vi "Begin.vi"(8 "error in":errorcluster) -> (0 "error out":errorcluster)   [LabVIEW 2019]
doc: "Called before other user functions, this VI can be used to open I/O refnums, load in file data, and do general program initialization. Notice that the <B>error out</B> terminal is simply used for data flow. Wiring it to other structures or subVIs ensures that this VI runs first."
uses:
  <vilib>/Rock Robotics/WPI/DriverStation/WPI_DriverStationRobotMode2.ctl
  <vilib>/Rock Robotics/WPI/Joystick/WPI_JoystickDeviceEnum.ctl
  <vilib>/Rock Robotics/SystemInterfaces/DIO/FPGA_DIOPWMChannel.ctl
  <vilib>/Rock Robotics/WPI/SafetyOutput/WPI_SafetyOutputConfigMenu.ctl
  <vilib>/Rock Robotics/WPI/Solenoid/WPI_SolenoidChannel.ctl
  <vilib>/Rock Robotics/SystemInterfaces/i2clib/i2c_bus.ctl
  <vilib>/Rock Robotics/WPI/Solenoid/WPI_SolenoidValue.ctl
  Robot Global Data.vi
  <vilib>/Rock Robotics/WPI/RobotDrive/WPI_RobotDriveOpen2MotorWithExistingMotors.vi
  <vilib>/Rock Robotics/WPI/MotorControl/WPI_MotorControlOpen SPARK.vi
  <vilib>/Rock Robotics/WPI/Solenoid/WPI_SolenoidOpenDouble.vi
  <vilib>/Rock Robotics/WPI/Solenoid/WPI_SolenoidSetEnum.vi
  <vilib>/Rock Robotics/Network Tables/NT Write Number.vi
  <vilib>/Rock Robotics/Network Tables/NT Write Boolean Array.vi
  <vilib>/Rock Robotics/Network Tables/NT Write Numeric Array.vi
panel:
  in  "Blue Calibration":cluster{"R":dbl, "G":dbl, "B":dbl}={"R"=0.143, "G"=0.427, "B"=0.429}
  in  "Green Calibration":cluster{"R":dbl, "G":dbl, "B":dbl}={"R"=0.197, "G"=0.561, "B"=0.24}
  in  "Red Calibration":cluster{"R":dbl, "G":dbl, "B":dbl}={"R"=0.561, "G"=0.323, "B"=0.114}
  in  "Yellow Calibration":cluster{"R":dbl, "G":dbl, "B":dbl}={"R"=0.361, "G"=0.524, "B"=0.113}
  in  "Calibration Time (sec)":u32=4
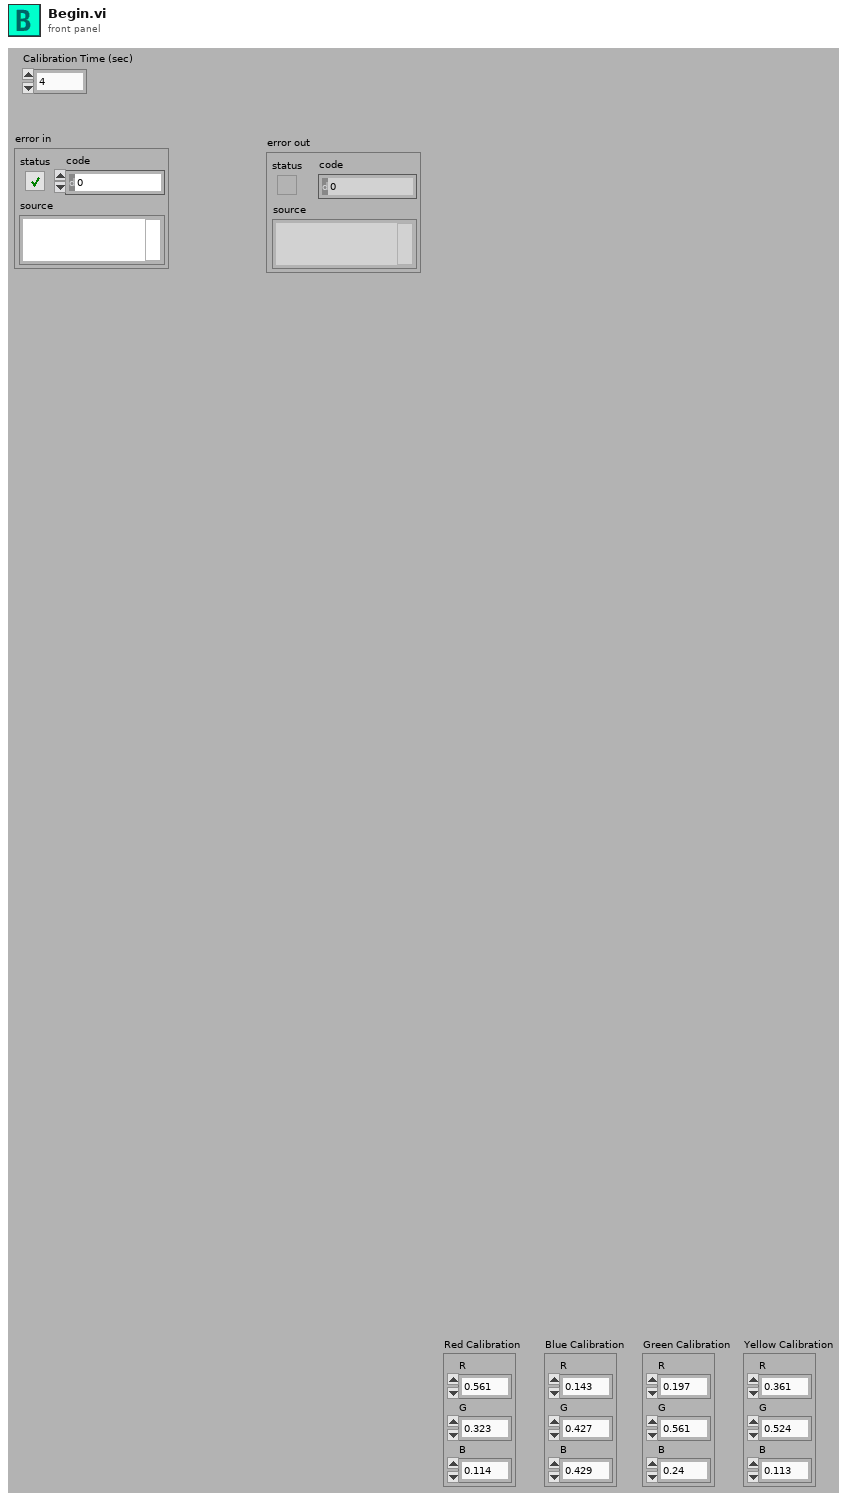
[diagram p1: front panel]
types:
  T1 = typedef "WPI_SolenoidChannel.ctl" = enum8{"Solenoid 0", "Solenoid 1", "Solenoid 2", "Solenoid 3", "Solenoid 4", "Solenoid 5", "Solenoid 6", "Solenoid 7", "Invalid"}
  T2 = typedef "WPI_SolenoidValue.ctl" = enum16{"Off", "On", "Forward", "Reverse"}
  T3 = typedef "WPI_SafetyOutputConfigMenu.ctl" = enum16{"Enable", "Disable"}
  T4 = typedef "i2c_bus.ctl" = enum16{"I2C On-Board", "I2C MXP", "Invalid"}
  T5 = typedef "FPGA_DIOPWMChannel.ctl" = enum8{"PWM 0", "PWM 1", "PWM 2", "PWM 3", "PWM 4", "PWM 5", "PWM 6", "PWM 7", "PWM 8", "PWM 9", "PWM MXP 0", "PWM MXP 1", "PWM MXP 2", "PWM MXP 3", "PWM MXP 4", "PWM MXP 5", "PWM MXP 6", "PWM MXP 7", "PWM MXP 8", "PWM MXP 9", "Invalid"}
  T6 = typedef "WPI_JoystickDeviceEnum.ctl" = enum16{"USB 0", "USB 1", "USB 2", "USB 3", "USB 4", "USB 5"}
  T7 = typedef "WPI_DriverStationRobotMode2.ctl" = enum16{"Autonomous Disabled", "Autonomous Enabled", "Teleop Disabled", "Teleop Enabled", "Disconnected", "Finish", "Test Disabled", "Test Enabled", "Emergency Stopped"}
  T8 = typedef "WPI_JoystickDevRef.ctl" = cluster{"Device":T6}
  T9 = typedef "WPI_MotorControlDeviceRef.ctl" = cluster{"DeviceStatus":errorcluster, "Type":T10, "PWM":cluster{"PWM Channel":T5, "DeadBand":T11}, "CAN":cluster{"Device Number":u8, "SetOutput VI Ref":variant, "GetOutput VI Ref":variant, "Enable VI Ref":variant, "Disable VI Ref":variant, "Data":variant}, "Invert":bool, "DIO PWM":cluster{"PWM \"Enable\" Channel":T5, "DIOChannel":T12, "PWM Rate":dbl}}
  T10 = typedef "WPI_MotorControlType.ctl" = enum16{"PWM", "CAN", "DIO PWM"}
  T11 = typedef "WPI_PWMDeadband.ctl" = cluster{"Name":string, "maxPositivePwm":i32, "minPositivePwm":i32, "centerPwm":i32, "maxNegativePwm":i32, "minNegativePwm":i32, "angularRange":u16}
  T12 = typedef "FPGA_DIOChannel.ctl" = enum8{"DIO 0", "DIO 1", "DIO 2", "DIO 3", "DIO 4", "DIO 5", "DIO 6", "DIO 7", "DIO 8", "DIO 9", "DIO MXP 0", "DIO MXP 1", "DIO MXP 2", "DIO MXP 3", "DIO MXP 4", "DIO MXP 5", "DIO MXP 6", "DIO MXP 7", "DIO MXP 8", "DIO MXP 9", "DIO MXP 10", "DIO MXP 11", "DIO MXP 12", "DIO MXP 13", "DIO MXP 14", "DIO MXP 15", "SPI Port CS1", "SPI Port CS2", "SPI Port CS3", "SPI Port MISO", "SPI Port MOSI", "Invalid"}
  T13 = typedef "WPI_RobotDriveDevRef.ctl" = cluster{"DevStatus":errorcluster, "Motors[]":T9[], "Square Inputs":bool, "Max Output":dbl}
  T14 = typedef "ADIS 16448 HW Configuration.ctl" = cluster{"SPI Clock Rate (Hz)":dbl, "IMU SPI Mode (3)":T15, "IMU Reset Pin":T12, "IMU SPI Bus":T16, "IMU Data Ready Pin":T12, "Stall Config":cluster{"Pow2BytesPerRead":u8, "StallTicks":u16, "CsToSclkTicks":u8}, "IMU Status LED Pin":T12}
  T15 = typedef "WPI_SPIMode.ctl" = enum16{"Mode 0 (Clk Idle Low,Sample on Leading)", "Mode 1 (Clk Idle Low,Sample on Trailing)", "Mode 2 (Clk Idle High,Sample on Leading)", "Mode 3 (Clk Idle High,Sample on Trailing)"}
  T16 = typedef "spi_bus.ctl" = enum16{"SPI On-Board, CS0", "SPI On-Board, CS1", "SPI On-Board, CS2", "SPI On-Board, CS3", "SPI MXP", "Invalid"}
  T17 = typedef "Color Sensor V3 DevRef.ctl" = cluster{"I2CDevRef":T18}
  T18 = typedef "WPI_I2CDevRef.ctl" = cluster{"DevStatus":errorcluster, "Device Address":u8, "Handle":i32, "I2C Bus":T4}
  T19 = typedef "WPI_SolenoidDevRef.ctl" = cluster{"DevStatus":errorcluster, "Pneumatics Control Module":u8, "Forward Solenoid Channel":T1, "Reverse Solenoid Channel":T1}
  T20 = typedef "ADIS16448 Device Reference.ctl" = cluster{"DevStatus":errorcluster, "Hardware Config":T21, "Calibration Complete":refnum<notifier>, "Status FIFO":refnum<k33>, "Last Value Reference":refnum<data-value>, "Sychronous Process VI":T22, "Cmd FIFO":refnum<k33>, "Source":T23, "Data FIFO":refnum<k33>, "IMU Status LED Pin":T12, "Calibration Time":u32}
  T21 = typedef "ADIS16448 Hardware Configuration.ctl" = cluster{"SPI Clock Rate (Hz)":dbl, "IMU SPI Mode (3)":T15, "IMU Reset Pin":T12, "IMU SPI Bus":T16, "IMU Data Ready Pin":T12, "Stall Config":cluster{"Pow2BytesPerRead":u8, "StallTicks":u16, "CsToSclkTicks":u8}, "IMU Status LED Pin":T12}
  T22 = typedef "ADIS16448 Process.ctl" = refnum<vi>
  T23 = typedef "FPGA_CounterEncoderSourceConvertionLVSourceType.ctl" = cluster{"DevStatus":errorcluster, "AnalogTriggerMode?":bool, "DigitalMode":cluster{"DIO Channel":T24}, "AnalogTriggerMode":cluster{"AnalogTriggerIndex":T25, "OutputType":T26}}
  T24 = typedef "FPGA_DIODigitalSourceChannel.ctl" = enum8{"DIO 0", "DIO 1", "DIO 2", "DIO 3", "DIO 4", "DIO 5", "DIO 6", "DIO 7", "DIO 8", "DIO 9", "DIO MXP 0", "DIO MXP 1", "DIO MXP 2", "DIO MXP 3", "DIO MXP 4", "DIO MXP 5", "DIO MXP 6", "DIO MXP 7", "DIO MXP 8", "DIO MXP 9", "DIO MXP 10", "DIO MXP 11", "DIO MXP 12", "DIO MXP 13", "DIO MXP 14", "DIO MXP 15", "SPI Port CS1", "SPI Port CS2", "SPI Port CS3", "SPI Port MISO", "SPI Port MOSI", "Disabled"}
  T25 = typedef "FPGA_AnalogTriggerIndex.ctl" = enum8{"Trig 0", "Trig 1", "Trig 2", "Trig 3", "Trig 4", "Trig 5", "Trig 6", "Trig 7", "Invalid"}
  T26 = typedef "FPGA_AnalogTriggerOutType.ctl" = enum16{"InWindow", "TriggerState", "Rising", "Falling"}
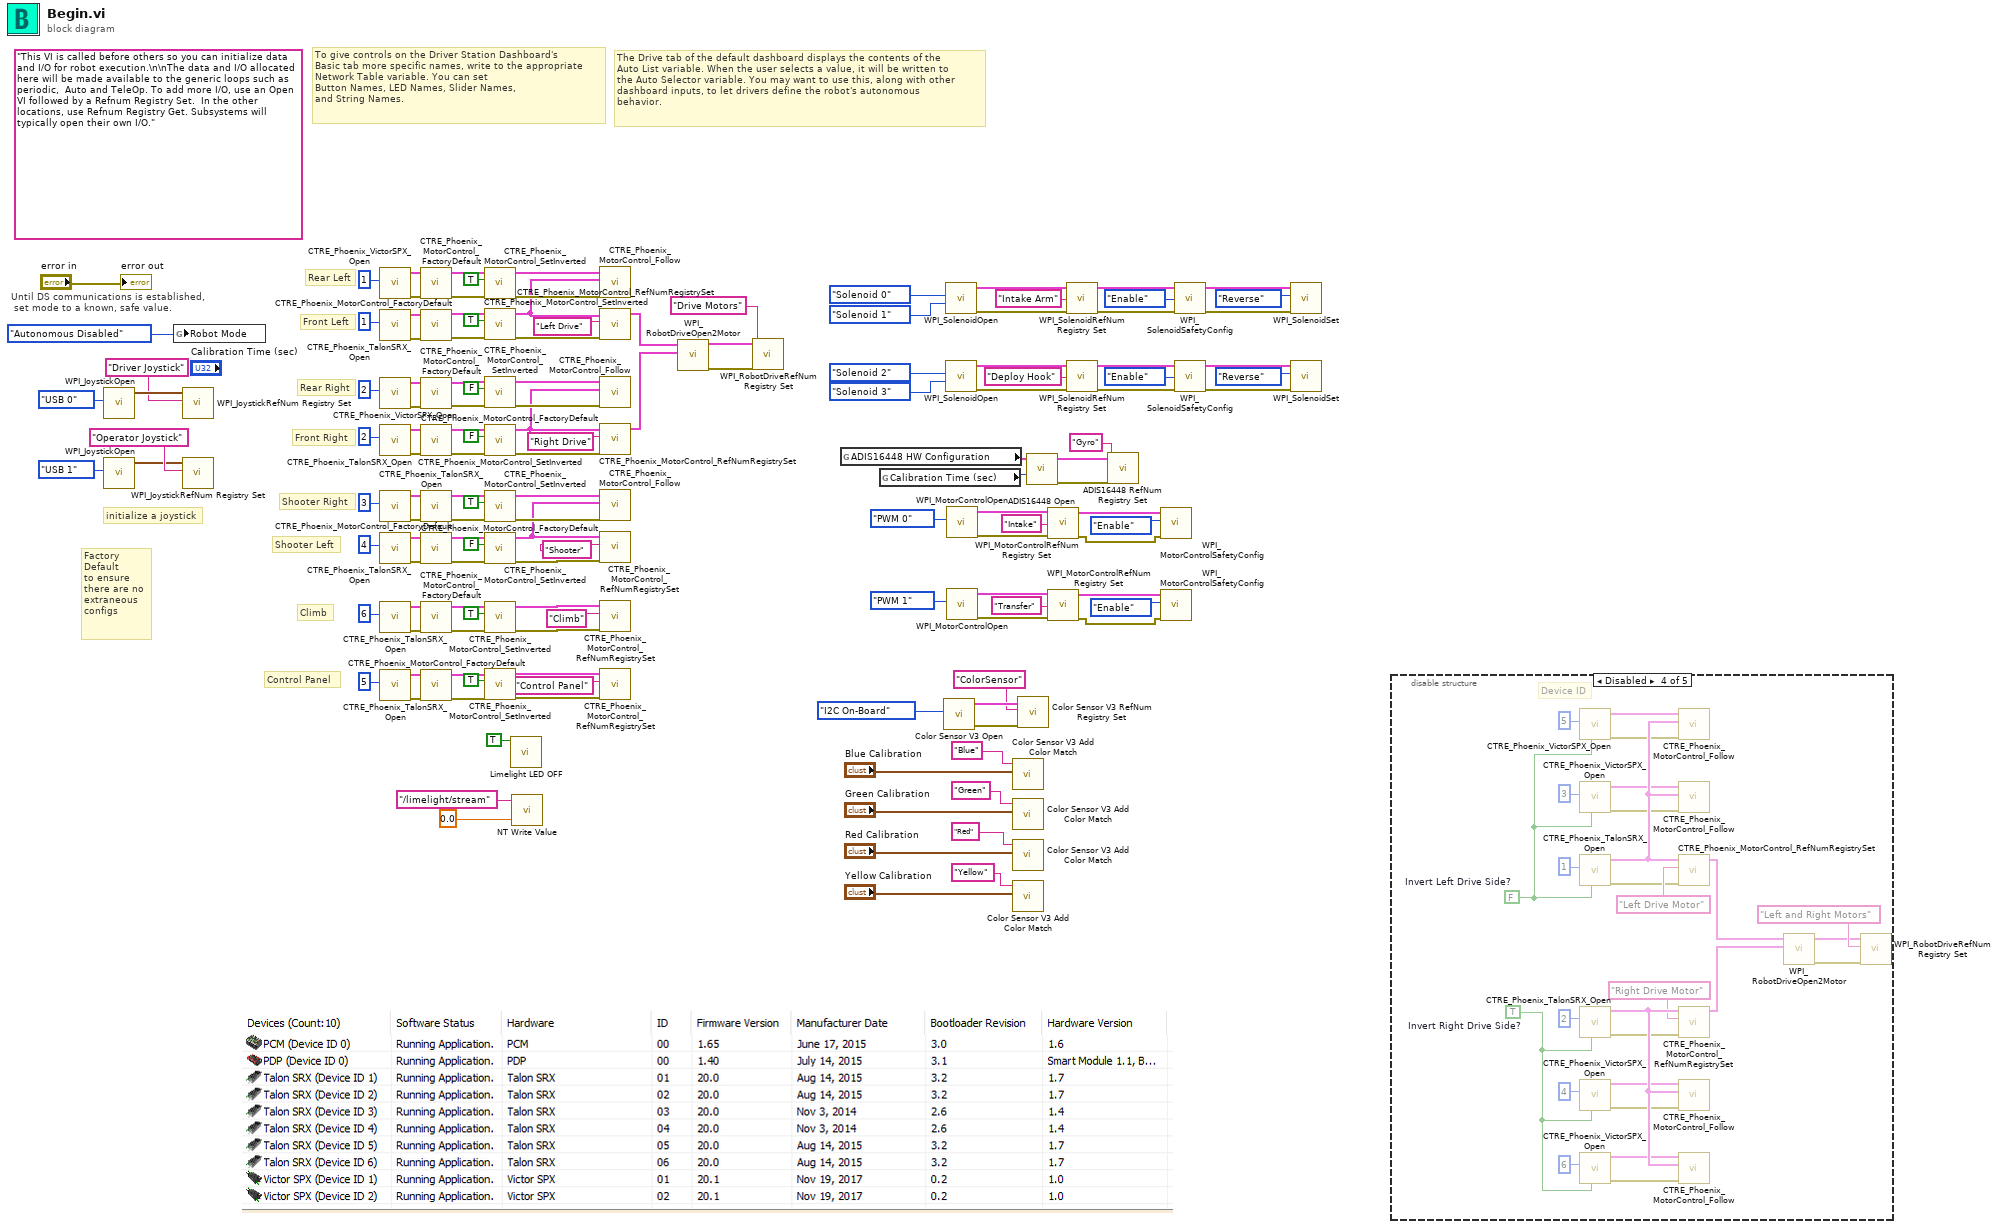
[diagram p0: block diagram]
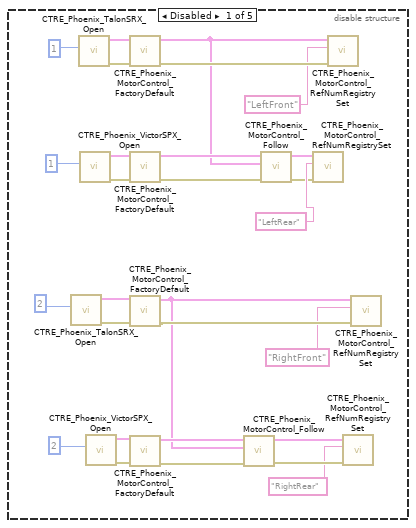
[diagram p2: hidden frame]
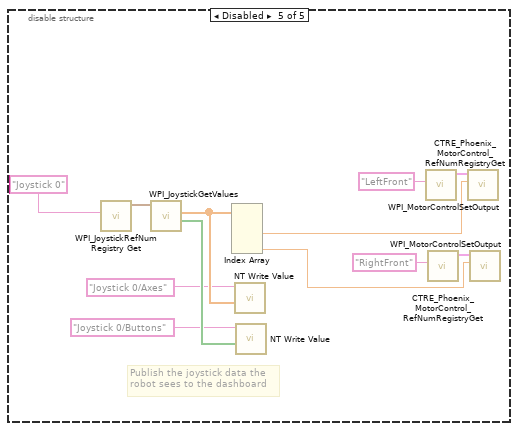
[diagram p5: hidden frame]
diagram:
  (unwired) "This VI is called before others so you can initialize data and I/O for robot execution.\n\nThe data and I/O allocated here will be made available to the generic loops such as periodic,  Auto and TeleOp. To add more I/O, use an Open VI followed by a Refnum Registry Set.  In the other locations, use Refnum Registry Get. Subsystems will typically open their own I/O."
  # "Climb"
  # "Control Panel"
  # "The Drive tab of the default dashboard displays the contents of the\nAuto List variable. When the user selects a value, it will be written to\nthe Auto Selector variable. You may want to use this, along with other\ndashboard inputs, to let drivers define the robot's autonomous\nbehavior."
  # "To give controls on the Driver Station Dashboard's\nBasic tab more specific names, write to the appropriate\nNetwork Table variable. You can set\nButton Names, LED Names, Slider Names,\nand String Names."
  # "Shooter Left"
  # "Shooter Right"
  # "Factory \nDefault \nto ensure \nthere are no \nextraneous \nconfigs"
  # "Front Right"
  # "Front Left"
  # "Rear Right"
  # "Rear Left"
  # "initialize a joystick"
  # "Until DS communications is established,\n set mode to a known, safe value."
  n1 = call <vilib>:"WPI_JoystickOpen.vi"("JoystickDevice"=WPI_JoystickDeviceEnum."USB 0") -> ("JoystickDevRef"=w121:T8)  [unwired: 10 in]
  n2 = call <vilib>:"WPI_JoystickOpen.vi"("JoystickDevice"=WPI_JoystickDeviceEnum."USB 1") -> ("JoystickDevRef"=w136:T8)  [unwired: 10 in]
  n3 = global write "Robot Global Data.vi" "Robot Mode"(WPI_DriverStationRobotMode2."Autonomous Disabled" ("Robot Mode")) -> ()
  n4 = call <vilib>:"WPI_JoystickRefNum Registry Set.vi"("refnum name"="Driver Joystick", "JoystickDevRef"=w121) -> ()  [unwired: 8 in, 2 out]
  n5 = call <vilib>:"WPI_JoystickRefNum Registry Set.vi"("refnum name"="Operator Joystick", "JoystickDevRef"=w136) -> ()  [unwired: 8 in, 2 out]
  n6 = call <vilib>:"CTRE_Phoenix_VictorSPX_Open.vi"("Device Number"=u8 1) -> ("error out"=w119:errorcluster, "CAN Talon SRX Ref"=w118:T9)  [unwired: 9 in]
  n7 = call <vilib>:"CTRE_Phoenix_TalonSRX_Open.vi"("Device Number"=u8 1) -> ("error out"=w116:errorcluster, "CAN Talon SRX Ref"=w117:T9)  [unwired: 9 in]
  n8 = call <vilib>:"CTRE_Phoenix_VictorSPX_Open.vi"("Device Number"=u8 2) -> ("error out"=w115:errorcluster, "CAN Talon SRX Ref"=w114:T9)  [unwired: 9 in]
  n9 = call <vilib>:"CTRE_Phoenix_TalonSRX_Open.vi"("Device Number"=u8 2) -> ("error out"=w113:errorcluster, "CAN Talon SRX Ref"=w112:T9)  [unwired: 9 in]
  n10 = call <vilib>:"CTRE_Phoenix_TalonSRX_Open.vi"("Device Number"=u8 3) -> ("error out"=w74:errorcluster, "CAN Talon SRX Ref"=w73:T9)  [unwired: 9 in]
  n11 = call <vilib>:"CTRE_Phoenix_TalonSRX_Open.vi"("Device Number"=u8 4) -> ("error out"=w72:errorcluster, "CAN Talon SRX Ref"=w71:T9)  [unwired: 9 in]
  n12 = call <vilib>:"CTRE_Phoenix_TalonSRX_Open.vi"("Device Number"=u8 6) -> ("error out"=w13:errorcluster, "CAN Talon SRX Ref"=w12:T9)  [unwired: 9 in]
  n13 = call <vilib>:"CTRE_Phoenix_TalonSRX_Open.vi"("Device Number"=u8 5) -> ("error out"=w47:errorcluster, "CAN Talon SRX Ref"=w46:T9)  [unwired: 9 in]
  n14 = call <vilib>:"CTRE_Phoenix_MotorControl_FactoryDefault.vi"("error in"=w119, "PhoenixMotorControlDevRef"=w118) -> ("error out"=w110:errorcluster, "PhoenixMotorControlDevRef"=w109:T9)  [unwired: 8 in]
  n15 = call <vilib>:"CTRE_Phoenix_MotorControl_FactoryDefault.vi"("error in"=w116, "PhoenixMotorControlDevRef"=w117) -> ("error out"=w104:errorcluster, "PhoenixMotorControlDevRef"=w105:T9)  [unwired: 8 in]
  n16 = call <vilib>:"CTRE_Phoenix_MotorControl_FactoryDefault.vi"("error in"=w115, "PhoenixMotorControlDevRef"=w114) -> ("error out"=w100:errorcluster, "PhoenixMotorControlDevRef"=w99:T9)  [unwired: 8 in]
  n17 = call <vilib>:"CTRE_Phoenix_MotorControl_FactoryDefault.vi"("error in"=w113, "PhoenixMotorControlDevRef"=w112) -> ("error out"=w95:errorcluster, "PhoenixMotorControlDevRef"=w94:T9)  [unwired: 8 in]
  n18 = call <vilib>:"CTRE_Phoenix_MotorControl_FactoryDefault.vi"("error in"=w74, "PhoenixMotorControlDevRef"=w73) -> ("error out"=w68:errorcluster, "PhoenixMotorControlDevRef"=w69:T9)  [unwired: 8 in]
  n19 = call <vilib>:"CTRE_Phoenix_MotorControl_FactoryDefault.vi"("error in"=w72, "PhoenixMotorControlDevRef"=w71) -> ("error out"=w63:errorcluster, "PhoenixMotorControlDevRef"=w64:T9)  [unwired: 8 in]
  n20 = call <vilib>:"CTRE_Phoenix_MotorControl_FactoryDefault.vi"("error in"=w13, "PhoenixMotorControlDevRef"=w12) -> ("error out"=w9:errorcluster, "PhoenixMotorControlDevRef"=w10:T9)  [unwired: 8 in]
  n21 = call <vilib>:"CTRE_Phoenix_MotorControl_FactoryDefault.vi"("error in"=w47, "PhoenixMotorControlDevRef"=w46) -> ("error out"=w43:errorcluster, "PhoenixMotorControlDevRef"=w44:T9)  [unwired: 8 in]
  n22 = call <vilib>:"CTRE_Phoenix_MotorControl_SetInverted.vi"("error in (no error)"=w110, "Invert?"=TRUE, "PhoenixMotorControlDevRef"=w109) -> ("error out"=w107:errorcluster, "PhoenixMotorControlDevRef"=w108:T9)  [unwired: 7 in]
  n23 = call <vilib>:"CTRE_Phoenix_MotorControl_SetInverted.vi"("error in (no error)"=w104, "Invert?"=TRUE, "PhoenixMotorControlDevRef"=w105) -> ("error out"=w103:errorcluster, "PhoenixMotorControlDevRef"=w102:T9)  [unwired: 7 in]
  n24 = call <vilib>:"CTRE_Phoenix_MotorControl_SetInverted.vi"("error in (no error)"=w100, "Invert?"=FALSE, "PhoenixMotorControlDevRef"=w99) -> ("error out"=w97:errorcluster, "PhoenixMotorControlDevRef"=w98:T9)  [unwired: 7 in]
  n25 = call <vilib>:"CTRE_Phoenix_MotorControl_SetInverted.vi"("error in (no error)"=w95, "Invert?"=FALSE, "PhoenixMotorControlDevRef"=w94) -> ("error out"=w92:errorcluster, "PhoenixMotorControlDevRef"=w93:T9)  [unwired: 7 in]
  n26 = call <vilib>:"CTRE_Phoenix_MotorControl_SetInverted.vi"("error in (no error)"=w68, "Invert?"=TRUE, "PhoenixMotorControlDevRef"=w69) -> ("error out"=w67:errorcluster, "PhoenixMotorControlDevRef"=w66:T9)  [unwired: 7 in]
  n27 = call <vilib>:"CTRE_Phoenix_MotorControl_SetInverted.vi"("error in (no error)"=w63, "Invert?"=FALSE, "PhoenixMotorControlDevRef"=w64) -> ("error out"=w62:errorcluster, "PhoenixMotorControlDevRef"=w61:T9)  [unwired: 7 in]
  n28 = call <vilib>:"CTRE_Phoenix_MotorControl_SetInverted.vi"("error in (no error)"=w9, "Invert?"=TRUE, "PhoenixMotorControlDevRef"=w10) -> ("error out"=w8:errorcluster, "PhoenixMotorControlDevRef"=w7:T9)  [unwired: 7 in]
  n29 = call <vilib>:"CTRE_Phoenix_MotorControl_SetInverted.vi"("error in (no error)"=w43, "Invert?"=TRUE, "PhoenixMotorControlDevRef"=w44) -> ("error out"=w42:errorcluster, "PhoenixMotorControlDevRef"=w41:T9)  [unwired: 7 in]
  n30 = call "Limelight LED OFF.vi"("D Select  8"=TRUE) -> ()  [unwired: 11 in]
  n31 = call-poly <vilib>:"NT Write Value.vi"("Numeric"=0.0, "Name"="/limelight/stream") -> ()  [unwired: 9 in, 1 out]
  n32 = call <vilib>:"CTRE_Phoenix_MotorControl_Follow.vi"("error in (no error)"=w107, "Master Controller to Follow"=w102, "PhoenixMotorControlDevRef"=w108) -> ()  [unwired: 7 in, 2 out]
  n33 = call <vilib>:"CTRE_Phoenix_MotorControl_RefNumRegistrySet.vi"("error in (no error)"=w103, "refnum name"="Left Drive", "PhoenixMotorControlDevRef"=w102) -> ("PhoenixMotorControlDevRef"=w129:T9)  [unwired: 7 in, 1 out]
  n34 = call <vilib>:"CTRE_Phoenix_MotorControl_Follow.vi"("error in (no error)"=w97, "Master Controller to Follow"=w93, "PhoenixMotorControlDevRef"=w98) -> ()  [unwired: 7 in, 2 out]
  n35 = call <vilib>:"CTRE_Phoenix_MotorControl_RefNumRegistrySet.vi"("error in (no error)"=w92, "refnum name"="Right Drive", "PhoenixMotorControlDevRef"=w93) -> ("PhoenixMotorControlDevRef"=w128:T9)  [unwired: 7 in, 1 out]
  n36 = call <vilib>:"CTRE_Phoenix_MotorControl_Follow.vi"("error in (no error)"=w67, "Master Controller to Follow"=w61, "PhoenixMotorControlDevRef"=w66) -> ()  [unwired: 7 in, 2 out]
  n37 = call <vilib>:"CTRE_Phoenix_MotorControl_RefNumRegistrySet.vi"("error in (no error)"=w62, "refnum name"="Shooter", "PhoenixMotorControlDevRef"=w61) -> ()  [unwired: 7 in, 2 out]
  n38 = call <vilib>:"CTRE_Phoenix_MotorControl_RefNumRegistrySet.vi"("error in (no error)"=w8, "refnum name"="Climb", "PhoenixMotorControlDevRef"=w7) -> ()  [unwired: 7 in, 2 out]
  n39 = call <vilib>:"CTRE_Phoenix_MotorControl_RefNumRegistrySet.vi"("error in (no error)"=w42, "refnum name"="Control Panel", "PhoenixMotorControlDevRef"=w41) -> ()  [unwired: 7 in, 2 out]
  n40 = call-poly <vilib>:"WPI_RobotDriveOpen2Motor.vi"("Right Motor Dev Ref"=w128, "Left Motor Dev Ref"=w129) -> ("error out"=w124:errorcluster, "RobotDriveDevRef"=w125:T13)  [unwired: 8 in]
  n41 = call <vilib>:"WPI_RobotDriveRefNum Registry Set.vi"("error in (no error)"=w124, "refnum name"="Drive Motors", "RobotDriveDevRef"=w125) -> ()  [unwired: 7 in, 2 out]
  n42 = global read "Robot Global Data.vi" "ADIS16448 HW Configuration"() -> (w5:T14)
  n43 = global read "Robot Global Data.vi" "Calibration Time (sec)"() -> (w4:u32)
  n44 = call <vilib>:"Color Sensor V3 Open.vi"("I2C Bus"=i2c_bus."I2C On-Board") -> ("error out"=w38:errorcluster, "ColorSensorDevRef"=w39:T17)  [unwired: 9 in]
  n45 = call-poly <vilib>:"WPI_SolenoidOpen.vi"("Reverse Solenoid Channel"=WPI_SolenoidChannel."Solenoid 1" ("Solenoid Channel"), "Forward Solenoid Channel"=WPI_SolenoidChannel."Solenoid 0" ("Solenoid Channel")) -> ("error out"=w57:errorcluster, "SolenoidDevRef"=w60:T19)  [unwired: 8 in]
  n46 = call-poly <vilib>:"WPI_SolenoidOpen.vi"("Reverse Solenoid Channel"=WPI_SolenoidChannel."Solenoid 3" ("Solenoid Channel"), "Forward Solenoid Channel"=WPI_SolenoidChannel."Solenoid 2" ("Solenoid Channel")) -> ("error out"=w20:errorcluster, "SolenoidDevRef"=w17:T19)  [unwired: 8 in]
  n47 = call-poly <vilib>:"WPI_MotorControlOpen.vi"("PWM Channel"=FPGA_DIOPWMChannel."PWM 0") -> ("error out"=w86:errorcluster, "MotorControlDeviceRef"=w90:T9)  [unwired: 9 in]
  n48 = call-poly <vilib>:"WPI_MotorControlOpen.vi"("PWM Channel"=FPGA_DIOPWMChannel."PWM 1") -> ("error out"=w83:errorcluster, "MotorControlDeviceRef"=w79:T9)  [unwired: 9 in]
  n49 = call <vilib>:"Color Sensor V3 Add Color Match.vi"("Color"="Blue Calibration", "Name"="Blue") -> ()  [unwired: 10 in]
  n50 = call <vilib>:"Color Sensor V3 Add Color Match.vi"("Color"="Green Calibration", "Name"="Green") -> ()  [unwired: 10 in]
  n51 = call <vilib>:"Color Sensor V3 Add Color Match.vi"("Color"="Red Calibration", "Name"="Red") -> ()  [unwired: 10 in]
  n52 = call <vilib>:"Color Sensor V3 Add Color Match.vi"("Color"="Yellow Calibration", "Name"="Yellow") -> ()  [unwired: 10 in]
  n53 = call <vilib>:"Color Sensor V3 RefNum Registry Set.vi"("error in (no error)"=w38, "refnum name"="ColorSensor", "ColorSensorDevRef"=w39) -> ()  [unwired: 7 in, 2 out]
  n54 = call <vilib>:"ADIS16448 Open.vi"("Initial Calibration Time (sec)"=w4, "Hardware Config"=w5) -> ("error out"=w2:errorcluster, "ADIS16448DevRef"=w3:T20)  [unwired: 8 in]
  n55 = call <vilib>:"WPI_MotorControlRefNum Registry Set.vi"("error in (no error)"=w86, "refnum name"="Intake", "MotorControlDevRef"=w90) -> ("error out"=w85:errorcluster, "MotorControlDevRef"=w89:T9)  [unwired: 7 in]
  n56 = call <vilib>:"WPI_MotorControlRefNum Registry Set.vi"("error in (no error)"=w83, "refnum name"="Transfer", "MotorControlDevRef"=w79) -> ("error out"=w84:errorcluster, "MotorControlDevRef"=w80:T9)  [unwired: 7 in]
  n57 = call <vilib>:"WPI_SolenoidRefNum Registry Set.vi"("error in (no error)"=w57, "refnum name"="Intake Arm", "SolenoidDevRef"=w60) -> ("error out"=w56:errorcluster, "SolenoidDevRef"=w59:T19)  [unwired: 7 in]
  n58 = call <vilib>:"WPI_SolenoidRefNum Registry Set.vi"("error in (no error)"=w20, "refnum name"="Deploy Hook", "SolenoidDevRef"=w17) -> ("error out"=w21:errorcluster, "SolenoidDevRef"=w18:T19)  [unwired: 7 in]
  n59 = call <vilib>:"ADIS16448 RefNum Registry Set.vi"("error in (no error)"=w2, "refnum name"="Gyro", "ADIS16448DevRef"=w3) -> ()  [unwired: 7 in, 2 out]
  n60 = call <vilib>:"WPI_MotorControlSafetyConfig.vi"("error in (no error)"=w85, "mode"=WPI_SafetyOutputConfigMenu."Enable", "MotorControlDevRef"=w89) -> ()  [unwired: 7 in, 2 out]
  n61 = call <vilib>:"WPI_MotorControlSafetyConfig.vi"("error in (no error)"=w84, "mode"=WPI_SafetyOutputConfigMenu."Enable", "MotorControlDevRef"=w80) -> ()  [unwired: 7 in, 2 out]
  n62 = call <vilib>:"WPI_SolenoidSafetyConfig.vi"("error in (no error)"=w56, "mode"=WPI_SafetyOutputConfigMenu."Enable", "SolenoidDevRef"=w59) -> ("error out"=w55:errorcluster, "SolenoidDevRef"=w58:T19)  [unwired: 7 in]
  n63 = call <vilib>:"WPI_SolenoidSafetyConfig.vi"("error in (no error)"=w21, "mode"=WPI_SafetyOutputConfigMenu."Enable", "SolenoidDevRef"=w18) -> ("error out"=w22:errorcluster, "SolenoidDevRef"=w19:T19)  [unwired: 7 in]
  n64 = call-poly <vilib>:"WPI_SolenoidSet.vi"("error in (no error)"=w55, "Value"=WPI_SolenoidValue."Reverse", "SolenoidDevRef"=w58) -> ()  [unwired: 7 in, 2 out]
  n65 = call-poly <vilib>:"WPI_SolenoidSet.vi"("error in (no error)"=w22, "Value"=WPI_SolenoidValue."Reverse", "SolenoidDevRef"=w19) -> ()  [unwired: 7 in, 2 out]
  n66 = disable-structure shown="Disabled" {
    frame Disabled {
      n67 = call <vilib>:"CTRE_Phoenix_TalonSRX_Open.vi"("Device Number"=u8 2) -> ("error out"=w163:errorcluster, "CAN Talon SRX Ref"=w153:T9)  [unwired: 9 in]
      n68 = call <vilib>:"CTRE_Phoenix_TalonSRX_Open.vi"("Device Number"=u8 1) -> ("error out"=w161:errorcluster, "CAN Talon SRX Ref"=w151:T9)  [unwired: 9 in]
      n69 = call <vilib>:"CTRE_Phoenix_VictorSPX_Open.vi"("Device Number"=u8 1) -> ("error out"=w159:errorcluster, "CAN Talon SRX Ref"=w157:T9)  [unwired: 9 in]
      n70 = call <vilib>:"CTRE_Phoenix_VictorSPX_Open.vi"("Device Number"=u8 2) -> ("error out"=w165:errorcluster, "CAN Talon SRX Ref"=w155:T9)  [unwired: 9 in]
      n71 = call <vilib>:"CTRE_Phoenix_MotorControl_FactoryDefault.vi"("error in"=w161, "PhoenixMotorControlDevRef"=w151) -> ("error out"=w162:errorcluster, "PhoenixMotorControlDevRef"=w152:T9)  [unwired: 8 in]
      n72 = call <vilib>:"CTRE_Phoenix_MotorControl_FactoryDefault.vi"("error in"=w159, "PhoenixMotorControlDevRef"=w157) -> ("error out"=w160:errorcluster, "PhoenixMotorControlDevRef"=w158:T9)  [unwired: 8 in]
      n73 = call <vilib>:"CTRE_Phoenix_MotorControl_FactoryDefault.vi"("error in"=w163, "PhoenixMotorControlDevRef"=w153) -> ("error out"=w164:errorcluster, "PhoenixMotorControlDevRef"=w154:T9)  [unwired: 8 in]
      n74 = call <vilib>:"CTRE_Phoenix_MotorControl_FactoryDefault.vi"("error in"=w165, "PhoenixMotorControlDevRef"=w155) -> ("error out"=w166:errorcluster, "PhoenixMotorControlDevRef"=w156:T9)  [unwired: 8 in]
      n75 = call <vilib>:"CTRE_Phoenix_MotorControl_Follow.vi"("error in (no error)"=w166, "Master Controller to Follow"=w154, "PhoenixMotorControlDevRef"=w156) -> ("error out"=w149:errorcluster, "PhoenixMotorControlDevRef"=w150:T9)  [unwired: 7 in]
      n76 = call <vilib>:"CTRE_Phoenix_MotorControl_Follow.vi"("error in (no error)"=w160, "Master Controller to Follow"=w152, "PhoenixMotorControlDevRef"=w158) -> ("error out"=w141:errorcluster, "PhoenixMotorControlDevRef"=w142:T9)  [unwired: 7 in]
      n77 = call <vilib>:"CTRE_Phoenix_MotorControl_RefNumRegistrySet.vi"("error in (no error)"=w141, "refnum name"="LeftRear", "PhoenixMotorControlDevRef"=w142) -> ()  [unwired: 7 in, 2 out]
      n78 = call <vilib>:"CTRE_Phoenix_MotorControl_RefNumRegistrySet.vi"("error in (no error)"=w162, "refnum name"="LeftFront", "PhoenixMotorControlDevRef"=w152) -> ()  [unwired: 7 in, 2 out]
      n79 = call <vilib>:"CTRE_Phoenix_MotorControl_RefNumRegistrySet.vi"("error in (no error)"=w149, "refnum name"="RightRear", "PhoenixMotorControlDevRef"=w150) -> ()  [unwired: 7 in, 2 out]
      n80 = call <vilib>:"CTRE_Phoenix_MotorControl_RefNumRegistrySet.vi"("error in (no error)"=w164, "refnum name"="RightFront", "PhoenixMotorControlDevRef"=w154) -> ()  [unwired: 7 in, 2 out]
    }
    frame Enabled {
    }
    frame Disabled {
    }
    frame Disabled {
      w193 = FALSE  # Invert Left Drive Side?
      w192 = TRUE  # Invert Right Drive Side?
      # "Device ID"
      n81 = call <vilib>:"CTRE_Phoenix_VictorSPX_Open.vi"("Invert"=w193, "Device Number"=u8 5) -> ("error out"=w183:errorcluster, "CAN Talon SRX Ref"=w184:T9)  [unwired: 8 in]
      n82 = call <vilib>:"CTRE_Phoenix_VictorSPX_Open.vi"("Invert"=w193, "Device Number"=u8 3) -> ("error out"=w182:errorcluster, "CAN Talon SRX Ref"=w185:T9)  [unwired: 8 in]
      n83 = call <vilib>:"CTRE_Phoenix_TalonSRX_Open.vi"("Invert"=w193, "Device Number"=u8 1) -> ("error out"=w173:errorcluster, "CAN Talon SRX Ref"=w186:T9)  [unwired: 8 in]
      n84 = call <vilib>:"CTRE_Phoenix_TalonSRX_Open.vi"("Invert"=w192, "Device Number"=u8 2) -> ("error out"=w174:errorcluster, "CAN Talon SRX Ref"=w181:T9)  [unwired: 8 in]
      n85 = call <vilib>:"CTRE_Phoenix_VictorSPX_Open.vi"("Invert"=w192, "Device Number"=u8 4) -> ("error out"=w177:errorcluster, "CAN Talon SRX Ref"=w178:T9)  [unwired: 8 in]
      n86 = call <vilib>:"CTRE_Phoenix_VictorSPX_Open.vi"("Invert"=w192, "Device Number"=u8 6) -> ("error out"=w180:errorcluster, "CAN Talon SRX Ref"=w179:T9)  [unwired: 8 in]
      n87 = call <vilib>:"CTRE_Phoenix_MotorControl_Follow.vi"("error in (no error)"=w183, "Master Controller to Follow"=w186, "PhoenixMotorControlDevRef"=w184) -> ()  [unwired: 7 in, 2 out]
      n88 = call <vilib>:"CTRE_Phoenix_MotorControl_Follow.vi"("error in (no error)"=w182, "Master Controller to Follow"=w186, "PhoenixMotorControlDevRef"=w185) -> ()  [unwired: 7 in, 2 out]
      n89 = call <vilib>:"CTRE_Phoenix_MotorControl_RefNumRegistrySet.vi"("error in (no error)"=w173, "refnum name"="Left Drive Motor", "PhoenixMotorControlDevRef"=w186) -> ("PhoenixMotorControlDevRef"=w187:T9)  [unwired: 7 in, 1 out]
      n90 = call <vilib>:"CTRE_Phoenix_MotorControl_RefNumRegistrySet.vi"("error in (no error)"=w174, "refnum name"="Right Drive Motor", "PhoenixMotorControlDevRef"=w181) -> ("PhoenixMotorControlDevRef"=w188:T9)  [unwired: 7 in, 1 out]
      n91 = call <vilib>:"CTRE_Phoenix_MotorControl_Follow.vi"("error in (no error)"=w177, "Master Controller to Follow"=w181, "PhoenixMotorControlDevRef"=w178) -> ()  [unwired: 7 in, 2 out]
      n92 = call <vilib>:"CTRE_Phoenix_MotorControl_Follow.vi"("error in (no error)"=w180, "Master Controller to Follow"=w181, "PhoenixMotorControlDevRef"=w179) -> ()  [unwired: 7 in, 2 out]
      n93 = call-poly <vilib>:"WPI_RobotDriveOpen2Motor.vi"("Right Motor Dev Ref"=w188, "Left Motor Dev Ref"=w187) -> ("error out"=w189:errorcluster, "RobotDriveDevRef"=w190:T13)  [unwired: 8 in]
      n94 = call <vilib>:"WPI_RobotDriveRefNum Registry Set.vi"("error in (no error)"=w189, "refnum name"="Left and Right Motors", "RobotDriveDevRef"=w190) -> ()  [unwired: 7 in, 2 out]
    }
    frame Disabled {
      # "Publish the joystick data the\nrobot sees to the dashboard"
      n95 = call <vilib>:"WPI_JoystickRefNum Registry Get.vi"("refnum name"="Joystick 0") -> ("JoystickDevRef"=w195:T8)  [unwired: 1 in, 9 out]
      n96 = call <vilib>:"WPI_JoystickGetValues.vi"("JoystickDevRef"=w195) -> ("Buttons"=w199:bool[], "Axes"=w198:dbl[])  [unwired: 6 in, 3 out]
      n97 = Index Array(array=w198) -> (element #2=w202:dbl, element #4=w205:dbl)  [unwired: 4 in, 2 out]
      n98 = call-poly <vilib>:"NT Write Value.vi"("Numeric Array"=w198, "Name"="Joystick 0/Axes") -> ()  [unwired: 9 in, 1 out]
      n99 = call-poly <vilib>:"NT Write Value.vi"("Boolean Array"=w199, "Name"="Joystick 0/Buttons") -> ()  [unwired: 9 in, 1 out]
      n100 = call <vilib>:"CTRE_Phoenix_MotorControl_RefNumRegistryGet.vi"("refnum name"="LeftFront") -> ("PhoenixMotorControlDevRef"=w201:T9)  [unwired: 9 in, 1 out]
      n101 = call <vilib>:"CTRE_Phoenix_MotorControl_RefNumRegistryGet.vi"("refnum name"="RightFront") -> ("PhoenixMotorControlDevRef"=w204:T9)  [unwired: 9 in, 1 out]
      n102 = call <vilib>:"WPI_MotorControlSetOutput.vi"("Output"=w202, "MotorControlDevRef"=w201) -> ()  [unwired: 7 in, 3 out]
      n103 = call <vilib>:"WPI_MotorControlSetOutput.vi"("Output"=w205, "MotorControlDevRef"=w204) -> ()  [unwired: 7 in, 3 out]
    }
  }
  "error out" <- "error in"
